vi "Decimation.vi"(0 "data in":T1[](array[typedef])=[{"I"=0.0, "Q"=0.0, "overflow"=FALSE}, {"I"=0.0, "Q"=0.0, "overflow"=FALSE}], 9 "input valid":bool, 11 "acq in":refnum<class "niUSRP Rx DSP v2 FPGA.lvclass">) -> (4 "data out":T1[](array[typedef]), 10 "output valid":bool, 14 "ready for input":bool, 15 "acq out":refnum<class "niUSRP Rx DSP v2 FPGA.lvclass">)   [LabVIEW 2025, in "niUSRP Rx DSP v2 FPGA.lvclass"]
uses:
  niUSRP Rx DSP v2 FPGA.lvclass
  <instrlib>/_niInstr/DSP/v1/Shared/Public/IQ Data.ctl
  niUSRP Rx DSP v2 FPGA.lvclass/niUSRP Rx DSP v2 FPGA.ctl
  <vilib>/rvi/DataTransferAndStorage/Container/Common/niFpgaContainerExecOnDevCompGetState.vi
  <vilib>/rvi/Emulation/niFpgaEmulationIsFPGAContextNoSignature.vi
  <vilib>/rvi/DataTransferAndStorage/Container/Common/niFpgaContainerGetUniqueNameForEmu.vi
  <vilib>/rvi/Memory/Memory_Emulation/niFpgaMemoryEmulationCacheClearOnFirstRun.vi
  <vilib>/rvi/Memory/Memory_Emulation/nirvimemoryEmulationManagerCache_MakeExclusive.vi
  <vilib>/rvi/Memory/Memory_Emulation/niFpgaMemoryEmulationValidateCache.vi
  <vilib>/rvi/Memory/Memory_Emulation/nirvimemoryEmulationManagerCache_InsertValue.vi
  <vilib>/Utility/error.llb/Clear Errors.vi
  <vilib>/rvi/Memory/Memory_Emulation/nirvimemoryEmulationManagerCache_ReleaseExclusive.vi
  <vilib>/rvi/Memory/Memory_Emulation/nirvimemoryEmulationManagerCache_GetValue.vi
  <vilib>/rvi/Memory/Memory_Emulation/nirvimemoryEmulationManagerCache_SetValue.vi
  <vilib>/rvi/Emulation/niFpgaProcessEmulError.vi
  <vilib>/rvi/Emulation/niFpgaSctlEmulationGetInTimedLoop.vi
  <vilib>/rvi/DataTransferAndStorage/Container/XNode/niFpgaContainer.xnode
  <vilib>/rvi/DataTransferAndStorage/Register/Emulation/niFpgaRegisterEmulationRefIn.vi
  <instrlib>/_niInstr/DSP Control/Interface/v1/FPGA/Decimation/IQ 18-bit/Decimation Interface (IQ 18-bit).lvclass
  <instrlib>/_niInstr/Basic Elements/v1/FPGA/niInstr Basic Elements v1 FPGA.lvlib
  <instrlib>/_niInstr/DSP/v1/Shared/niInstr DSP v1 Shared.lvlib
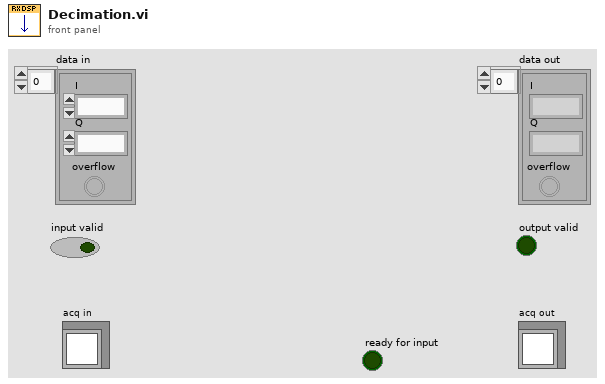
[diagram p1: front panel]
types:
  T1 = typedef "niInstr DSP v1 Shared.lvlib/IQ Data.ctl" = cluster{"I":fxp<+/-,18,1>, "Q":fxp<+/-,18,1>, "overflow":bool}
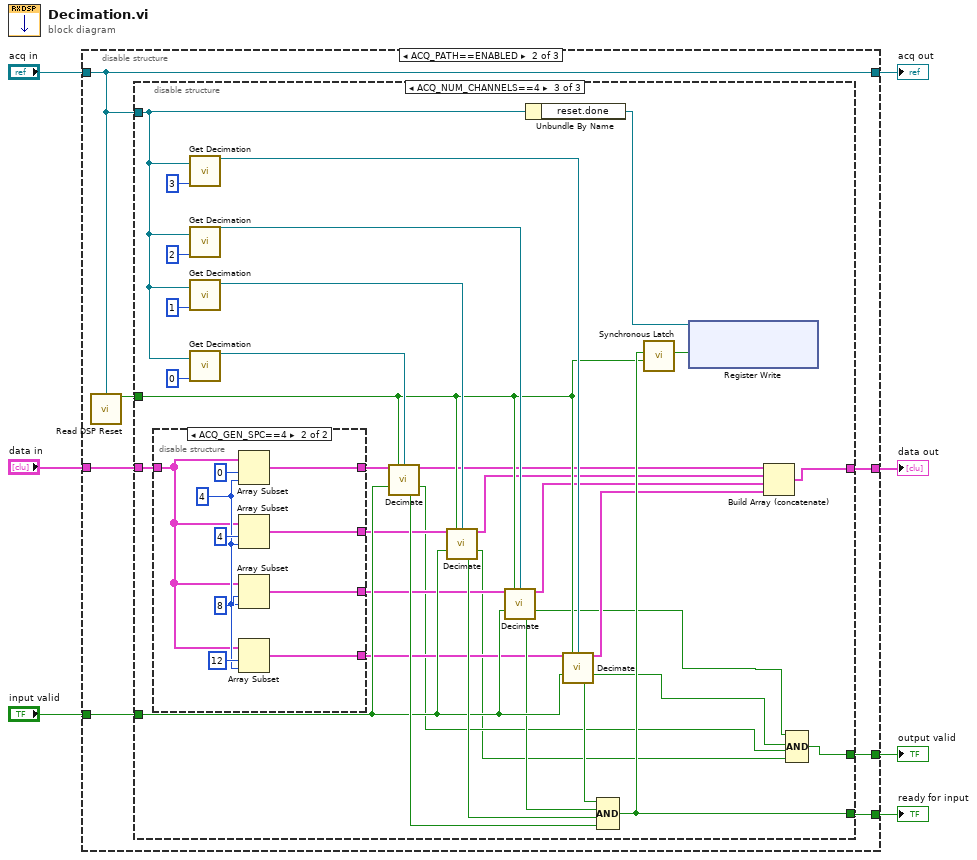
[diagram p0: block diagram]
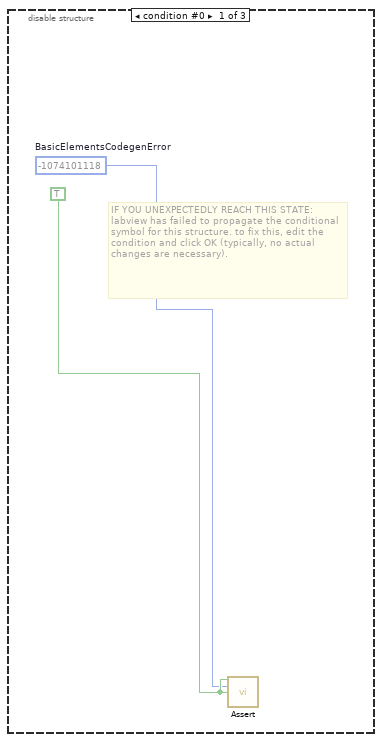
[diagram p2: hidden frame]
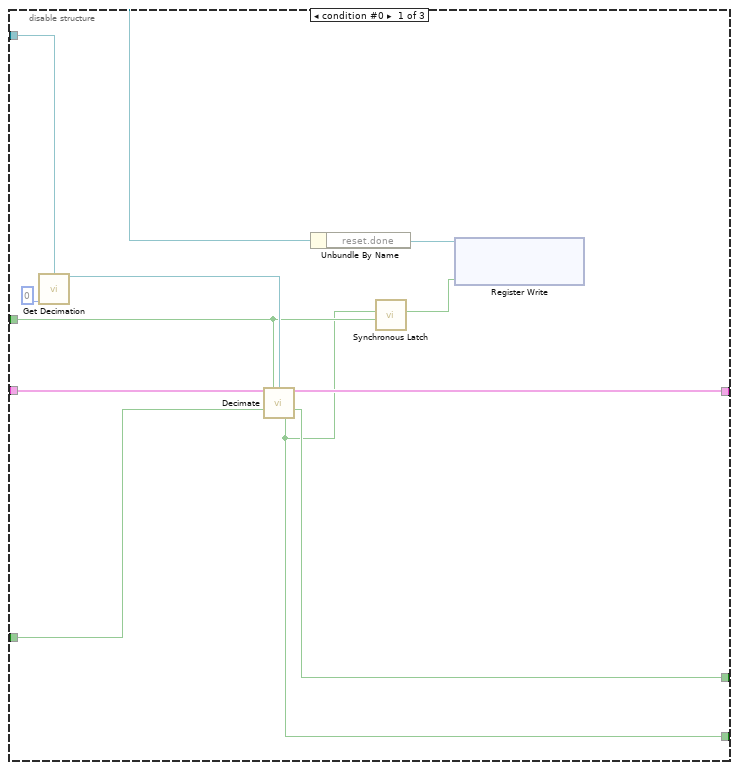
[diagram p3: hidden frame]
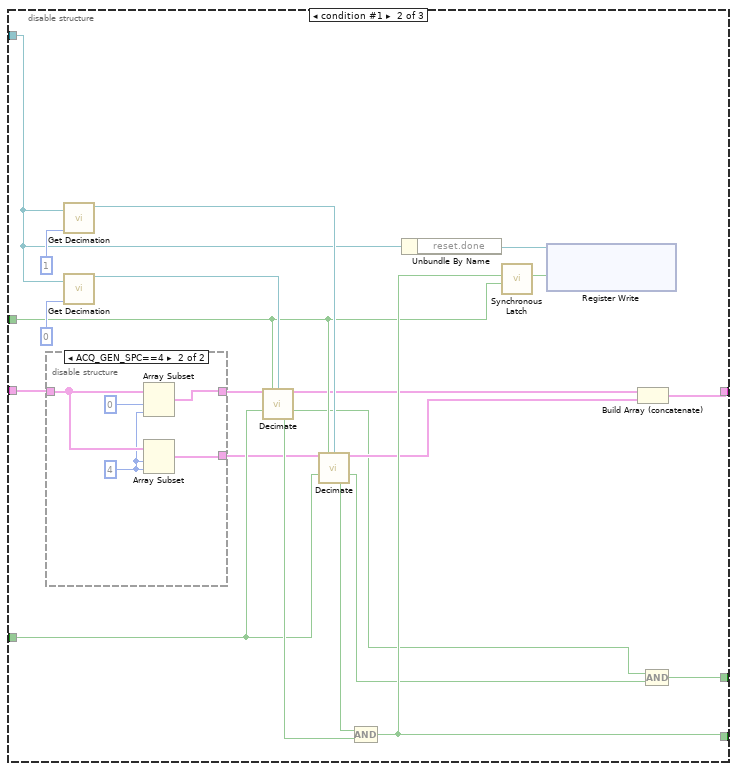
[diagram p4: hidden frame]
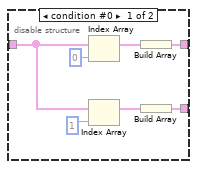
[diagram p5: hidden frame]
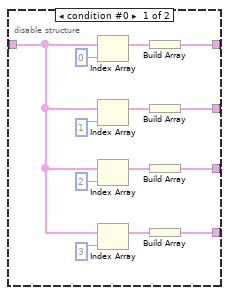
[diagram p6: hidden frame]
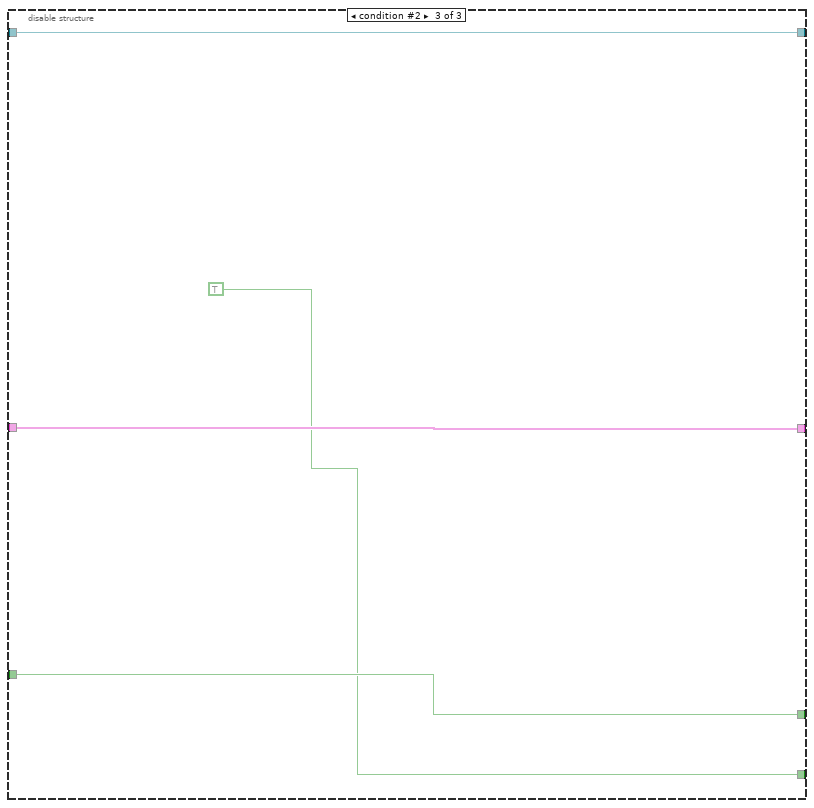
[diagram p7: hidden frame]
diagram:
  n1 = disable-structure shown="ACQ_PATH==ENABLED" {
    disable-tunnel: [_ w16 w118] -> w7
    disable-tunnel: [_ w11 w119] -> w6
    disable-tunnel: "data in" -> [_ w10 w118]
    disable-tunnel: "input valid" -> [_ w15 w119]
    disable-tunnel: "acq in" -> [_ w14 w120]
    disable-tunnel: [_ w14 w120] -> w3
    disable-tunnel: [_ w13 TRUE ("ready for input")] -> w2
    frame condition #0 {
      w9 = TRUE ("assert")
      w8 = -1074101118  # BasicElementsCodegenError
      # "IF YOU UNEXPECTEDLY REACH THIS STATE:\nlabview has failed to propagate the conditional symbol for this structure. to fix this, edit the condition and click OK (typically, no actual changes are necessary)."
      n2 = call <instrlib>:"Assert.vi"("assert"=w9, "error code"=w8, "enable show error"=w9) -> ()  [unwired: 13 in]
    }
    frame condition #1 (active) {
      n3 = call-dynamic "Read DSP Reset.vi"("acq"=w14) -> ("dsp reset"=w12:bool)  [unwired: 14 in]
      n4 = disable-structure shown="ACQ_NUM_CHANNELS==4" {
        disable-tunnel: [w27 w45 w90] -> w16
        disable-tunnel: w15 -> [w26 w38 w77]
        disable-tunnel: w14 -> [w24 w36 w80]
        disable-tunnel: [w17 w37 w83] -> w13
        disable-tunnel: w12 -> [w21 w35 w74]
        disable-tunnel: [w20 w44 w89] -> w11
        disable-tunnel: w10 -> [w18 w34 w73]
        frame condition #0 {
          n5 = call-dynamic "Get Decimation.vi"("acq in"=w24, "ch"=u8 0) -> ("decimation"=w25:refnum<class "Decimation Interface (IQ 18-bit).lvclass">)  [unwired: 13 in]
          n6 = call-dynamic "Decimate.vi"("data in"=w18, "reset"=w21, "decimation"=w25, "input valid"=w26) -> ("data out"=w27:T1[], "output valid"=w20:bool, "ready for input"=w17:bool)  [unwired: 8 in, 1 out]
          n7 = Unbundle By Name(w24) -> ("reset.done"=w23:refnum<k21>)
          n8 = call <instrlib>:"Synchronous Latch.vi"("clear"=w21, "set"=w17) -> ("out"=w22:bool)  [unwired: 9 in]
          n9 = xnode ("Register Write")("Data"=w22, "Register In"=w23) -> ()  [unwired: 1 out]
        }
        frame condition #1 {
          n10 = disable-structure shown="ACQ_GEN_SPC==4" {
            disable-tunnel: w34 -> [w51 w58]
            disable-tunnel: [w50 w59] -> w33
            disable-tunnel: [w49 w57] -> w32
            frame condition #0 {
              n11 = Index Array(array=w51, index=0) -> (element=w55:T1)
              n12 = Index Array(array=w51, index=1) -> (element=w53:T1)
              n13 = Build Array(w55) -> (w50:T1[])
              n14 = Build Array(w53) -> (w49:T1[])
            }
            frame condition #1 (active) {
              w56 = 4 ("length")
              n15 = Array Subset(array=w58, index=0, length=w56) -> (w59:T1[])
              n16 = Array Subset(array=w58, index=w56, length=w56) -> (w57:T1[])
            }
          }
          n17 = call-dynamic "Get Decimation.vi"("acq in"=w36, "ch"=u8 1) -> ("decimation"=w41:refnum<class "Decimation Interface (IQ 18-bit).lvclass">)  [unwired: 13 in]
          n18 = call-dynamic "Get Decimation.vi"("acq in"=w36, "ch"=u8 0) -> ("decimation"=w48:refnum<class "Decimation Interface (IQ 18-bit).lvclass">)  [unwired: 13 in]
          n19 = call-dynamic "Decimate.vi"("data in"=w33, "reset"=w35, "decimation"=w48, "input valid"=w38) -> ("data out"=w31:T1[], "output valid"=w29:bool, "ready for input"=w40:bool)  [unwired: 8 in, 1 out]
          n20 = call-dynamic "Decimate.vi"("data in"=w32, "reset"=w35, "decimation"=w41, "input valid"=w38) -> ("data out"=w30:T1[], "output valid"=w28:bool, "ready for input"=w39:bool)  [unwired: 8 in, 1 out]
          n21 = Compound Arithmetic op=AND(w39, w40) -> (w37:bool)
          n22 = Unbundle By Name(w36) -> ("reset.done"=w47:refnum<k21>)
          n23 = call <instrlib>:"Synchronous Latch.vi"("clear"=w35, "set"=w37) -> ("out"=w46:bool)  [unwired: 9 in]
          n24 = xnode ("Register Write")("Data"=w46, "Register In"=w47) -> ()  [unwired: 1 out]
          n25 = Build Array (concatenate)(w31, w30) -> (w45:T1[])
          n26 = Compound Arithmetic op=AND(w29, w28) -> (w44:bool)
        }
        frame condition #2 (active) {
          n27 = disable-structure shown="ACQ_GEN_SPC==4" {
            disable-tunnel: [w102 w110] -> w72
            disable-tunnel: [w101 w109] -> w71
            disable-tunnel: [w100 w108] -> w70
            disable-tunnel: w73 -> [w95 w111]
            disable-tunnel: [w94 w107] -> w69
            frame condition #0 {
              n28 = Index Array(array=w95, index=0) -> (element=w106:T1)
              n29 = Index Array(array=w95, index=1) -> (element=w104:T1)
              n30 = Index Array(array=w95, index=2) -> (element=w96:T1)
              n31 = Index Array(array=w95, index=3) -> (element=w98:T1)
              n32 = Build Array(w106) -> (w102:T1[])
              n33 = Build Array(w104) -> (w101:T1[])
              n34 = Build Array(w96) -> (w100:T1[])
              n35 = Build Array(w98) -> (w94:T1[])
            }
            frame condition #1 (active) {
              w112 = 4 ("length")
              n36 = Array Subset(array=w111, index=0, length=w112) -> (w110:T1[])
              n37 = Array Subset(array=w111, index=4, length=w112) -> (w109:T1[])
              n38 = Array Subset(array=w111, index=8, length=w112) -> (w108:T1[])
              n39 = Array Subset(array=w111, index=12, length=w112) -> (w107:T1[])
            }
          }
          n40 = call-dynamic "Get Decimation.vi"("acq in"=w80, "ch"=u8 3) -> ("decimation"=w78:refnum<class "Decimation Interface (IQ 18-bit).lvclass">)  [unwired: 13 in]
          n41 = call-dynamic "Get Decimation.vi"("acq in"=w80, "ch"=u8 2) -> ("decimation"=w79:refnum<class "Decimation Interface (IQ 18-bit).lvclass">)  [unwired: 13 in]
          n42 = call-dynamic "Get Decimation.vi"("acq in"=w80, "ch"=u8 1) -> ("decimation"=w86:refnum<class "Decimation Interface (IQ 18-bit).lvclass">)  [unwired: 13 in]
          n43 = call-dynamic "Get Decimation.vi"("acq in"=w80, "ch"=u8 0) -> ("decimation"=w93:refnum<class "Decimation Interface (IQ 18-bit).lvclass">)  [unwired: 13 in]
          n44 = call-dynamic "Decimate.vi"("data in"=w72, "reset"=w74, "decimation"=w93, "input valid"=w77) -> ("data out"=w68:T1[], "output valid"=w62:bool, "ready for input"=w85:bool)  [unwired: 8 in, 1 out]
          n45 = call-dynamic "Decimate.vi"("data in"=w71, "reset"=w74, "decimation"=w86, "input valid"=w77) -> ("data out"=w67:T1[], "output valid"=w61:bool, "ready for input"=w84:bool)  [unwired: 8 in, 1 out]
          n46 = call-dynamic "Decimate.vi"("data in"=w70, "reset"=w74, "decimation"=w79, "input valid"=w77) -> ("data out"=w66:T1[], "output valid"=w64:bool, "ready for input"=w76:bool)  [unwired: 8 in, 1 out]
          n47 = Unbundle By Name(w80) -> ("reset.done"=w92:refnum<k21>)
          n48 = call-dynamic "Decimate.vi"("data in"=w69, "reset"=w74, "decimation"=w78, "input valid"=w77) -> ("data out"=w65:T1[], "output valid"=w63:bool, "ready for input"=w75:bool)  [unwired: 8 in, 1 out]
          n49 = Compound Arithmetic op=AND(w75, w76, w84, w85) -> (w83:bool)
          n50 = call <instrlib>:"Synchronous Latch.vi"("clear"=w74, "set"=w83) -> ("out"=w91:bool)  [unwired: 9 in]
          n51 = xnode ("Register Write")("Data"=w91, "Register In"=w92) -> ()  [unwired: 1 out]
          n52 = Build Array (concatenate)(w68, w67, w66, w65) -> (w90:T1[])
          n53 = Compound Arithmetic op=AND(w64, w63, w62, w61) -> (w89:bool)
        }
      }
    }
    frame condition #2 {
    }
  }
  "data out" <- w7
  "output valid" <- w6
  "ready for input" <- w2
  "acq out" <- w3
